vi "instrumentProperties_channel_range.vi"(8 "error in (no error)":errorcluster, 11 "OSAchannel in":refnum<class "OSAchannel.lvclass">) -> (0 "error out":errorcluster, 1 "waveMax (cm^-1)":sgl, 2 "waveMin (cm^-1)":sgl, 3 "OSAchannel out":refnum<class "OSAchannel.lvclass">)   [LabVIEW 2010, in "OSAchannel.lvclass"]
uses:
  OSAchannel.lvclass
  FTSLib.dll
  OSA.lvclass
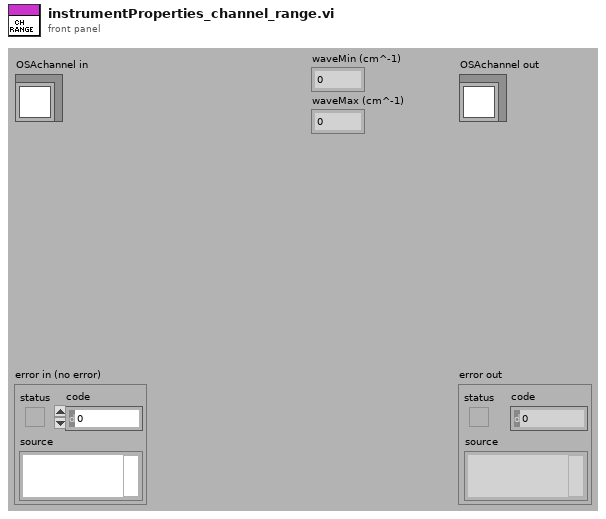
[diagram p1: front panel]
types:
  T1 = cluster{"waveMin (cm-1)":sgl, "waveMax (cm-1)":sgl, "gainOffset_auto":bool, "gain":i32, "gain levels nr":u16, "offset":i32, "offset max":u16, "damper available":bool, "damper active":bool, "amplifier type":i32, "detector type":i32, "channelIdx global":u16, "spectrIdx":u16, "waveMeter on":bool, "ref gainLevels rel.":refnum<data-value>}
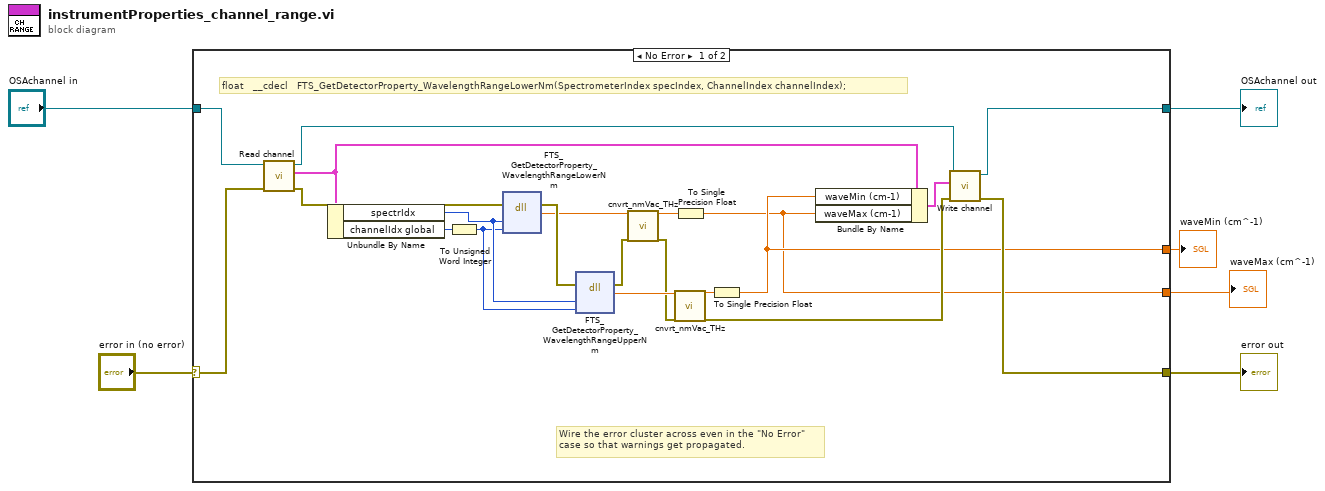
[diagram p0: block diagram]
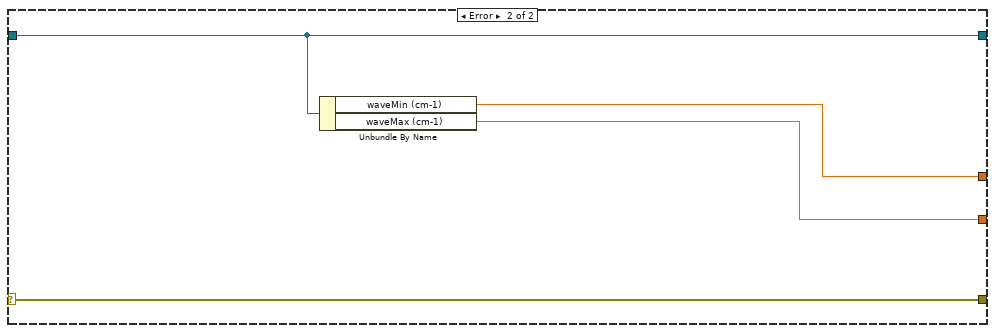
[diagram p2: hidden frame]
diagram:
  n1 = case shown="No Error" "error in (no error)" {
    selector: "error in (no error)" -> [w26 w31]
    tunnel: [w10 w31] -> w5
    tunnel: [w9 w30] -> w4
    tunnel: "OSAchannel in" -> [w27 w30]
    tunnel: [w7 w28] -> w2
    tunnel: [w8 w29] -> w3
    frame No Error {
      # "float\t\t\t__cdecl   FTS_GetDetectorProperty_WavelengthRangeLowerNm(SpectrometerIndex specIndex, ChannelIndex channelIndex);"
      # "Wire the error cluster across even in the \"No Error\"\ncase so that warnings get propagated."
      n2 = call "Read channel.vi"("error in (no error)"=w26, "OSAchannel in"=w27) -> ("error out"=w25:errorcluster, "channel"=w22:T1, "OSAchannel out"=w23:refnum<class "OSAchannel.lvclass">)  [unwired: 7 in]
      n3 = Unbundle By Name(w22) -> ("spectrIdx"=w20:u16, "channelIdx global"=w24:u16)
      n4 = To Unsigned Word Integer(number=w24) -> (unsigned 16bit integer=w19:u16)
      n5 = dll-call lib="FTSLib.dll" fn="FTS_GetDetectorProperty_WavelengthRangeLowerNm"(error in=w25, "spectrIdx"=w20, "channeldx"=w19) -> (error out=w21:errorcluster, "rangeLow_nm"=w17:sgl)  [unwired: 4 in, 1 out]
      n6 = dll-call lib="FTSLib.dll" fn="FTS_GetDetectorProperty_WavelengthRangeUpperNm"(error in=w21, "spectrIdx"=w20, "channeldx"=w19) -> (error out=w18:errorcluster, "rangeHigh_nm"=w15:sgl)  [unwired: 4 in, 1 out]
      n7 = call "cnvrt_nmVac_THz.vi"("nmVac"=w17, "error in (no error)"=w18) -> ("THz"=w16:dbl, "error out"=w13:errorcluster)  [unwired: 16 in]
      n8 = call "cnvrt_nmVac_THz.vi"("nmVac"=w15, "error in (no error)"=w13) -> ("THz"=w14:dbl, "error out"=w11:errorcluster)  [unwired: 16 in]
      n9 = To Single Precision Float(number=w16) -> (single precision float=w7:sgl)
      n10 = To Single Precision Float(number=w14) -> (single precision float=w8:sgl)
      n11 = Bundle By Name(cluster=w22, "waveMin (cm-1)"=w8, "waveMax (cm-1)"=w7) -> (w12:T1)
      n12 = call "Write channel.vi"("error in (no error)"=w11, "channel"=w12, "OSAchannel in"=w23) -> ("error out"=w10:errorcluster, "OSAchannel out"=w9:refnum<class "OSAchannel.lvclass">)  [unwired: 7 in]
    }
    frame Error {
      n13 = Unbundle By Name(w30) -> ("waveMin (cm-1)"=w29:sgl, "waveMax (cm-1)"=w28:sgl)
    }
  }
  "error out" <- w5
  "OSAchannel out" <- w4
  "waveMin (cm^-1)" <- w3
  "waveMax (cm^-1)" <- w2
